vi "Fetch Multi Eval Meas List Segment ES Flatness Subcarrier Index Results.vi"(8 "error in (no error)":errorcluster, 9 "Segment (1)":T3=1, 10 "Instance (1)":T4=1, 11 "VISA resource name":refnum<visa-resource-name>) -> (0 "error out":errorcluster, 1 "Subcarrier Index Results":T1, 2 "Reliability":T2, 3 "VISA resource name out":refnum<visa-resource-name>, 4 "Expired Statistics":i32, 5 "Out Of Tolerance":i32)   [LabVIEW 2020, in "Rohde&Schwarz CMWXP NR FR1 Measurement.lvlib"]
doc: "Return subcarrier indices of the equalizer spectrum flatness measurement for segment <no> in list mode. At these SC indices, the current minimum and maximum power of the equalizer coefficients have been detected within range 1 and range 2.\n\nAttribute:\nRSCMWXPNRFR1M_ATTR_FETCH_MULTI_EVAL_MEAS_LIST_SEGMENT_ES_FLATNESS_SUBCARRIER_INDEX_RESULTS\n\nRemote-control command:\nFETCh:NRSub:MEAS<i>:MEValuation:LIST:SEGMent<no>:ESFLatness:CURRent:SCINdex?"
uses:
  <instrlib>/Rohde&Schwarz CMWXP NR FR1 Measurement/Rohde&Schwarz CMWXP NR FR1 Measurement.lvlib
  <instrlib>/Rohde&Schwarz CMWXP NR FR1 Measurement/Private/_Instance.ctl
  <instrlib>/Rohde&Schwarz CMWXP NR FR1 Measurement/Private/_Segment.ctl
  <instrlib>/Rohde&Schwarz CMWXP NR FR1 Measurement/Private/_SegReliability.ctl
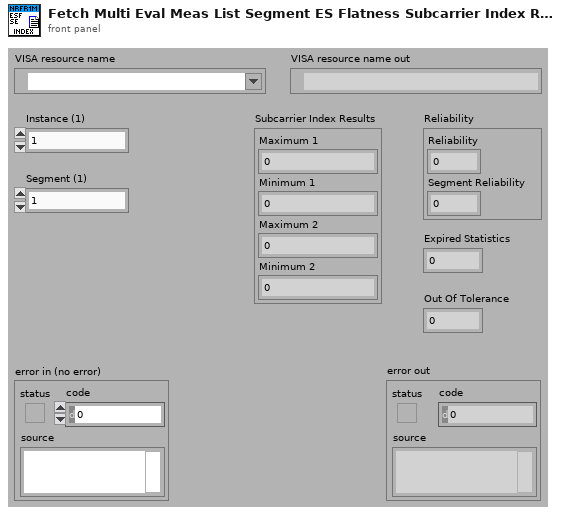
[diagram p1: front panel]
types:
  T1 = cluster{"Maximum 1":i32, "Minimum 1":i32, "Maximum 2":i32, "Minimum 2":i32}
  T2 = typedef "Rohde&Schwarz CMWXP NR FR1 Measurement.lvlib/_SegReliability.ctl" = cluster{"Reliability":i32, "Segment Reliability":i32}
  T3 = typedef "Rohde&Schwarz CMWXP NR FR1 Measurement.lvlib/_Segment.ctl" = i32
  T4 = typedef "Rohde&Schwarz CMWXP NR FR1 Measurement.lvlib/_Instance.ctl" = i32
  T5 = cluster{"Results[0]":i32, "Results[1]":i32, "Results[2]":i32, "Results[3]":i32}
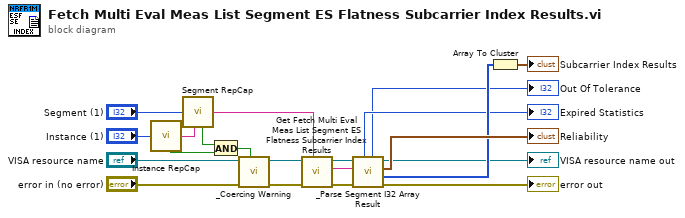
[diagram p0: block diagram]
diagram:
  n1 = call <instrlib>:"Instance RepCap.vi"("Instance In"="Instance (1)") -> ("In Range?"=w18:bool, "RepCap Identifier Out"=w17:string)  [unwired: 1 in]
  n2 = call <instrlib>:"Segment RepCap.vi"("Segment In"="Segment (1)", "RepCap String In (\"\")"=w17) -> ("In Range?"=w16:bool, "RepCap Identifier Out"=w15:string)
  n3 = And(x=w16, y=w18) -> (x .and. y?=w14:bool)
  n4 = call <instrlib>:"_Coercing Warning.vi"("In Range?"=w14, "error in (no error)"="error in (no error)", "VISA resource name"="VISA resource name") -> ("error out"=w11:errorcluster, "VISA resource name out"=w12:refnum<visa-resource-name>)  [unwired: 7 in]
  n5 = call "Get Fetch Multi Eval Meas List Segment ES Flatness Subcarrier Index Results"("Repeated Capabilities"=w15, "error in (no error)"=w11, "instrument handle"=w12) -> ("error out"=w8:errorcluster, "Fetch Multi Eval Meas List Segment ES Flatness Subcarrier Index Results"=w9:string, "instrument handle out"=w10:refnum<visa-resource-name>)  [unwired: 6 in]
  n6 = call <instrlib>:"_Parse Segment I32 Array Result.vi"("error in (no error)"=w8, "Input String"=w9, "VISA resource name"=w10) -> ("error out"=→"error out":errorcluster, "Results"=w5:i32[], "Reliability Results"=→"Reliability":T2, "VISA resource name out"=→"VISA resource name out":refnum<visa-resource-name>, "Out Of Tolerance"=→"Out Of Tolerance":i32, "Statistic Expired"=→"Expired Statistics":i32)  [unwired: 3 in]
  n7 = Array To Cluster(array=w5) -> (cluster=→"Subcarrier Index Results":T5)
